vi "strip_path_multiple.vi"(8 "error in (no error)":errorcluster, 10 "number of strips":i32=1, 11 "path in":path) -> (0 "error out":errorcluster, 3 "path out":path)   [LabVIEW 2010]
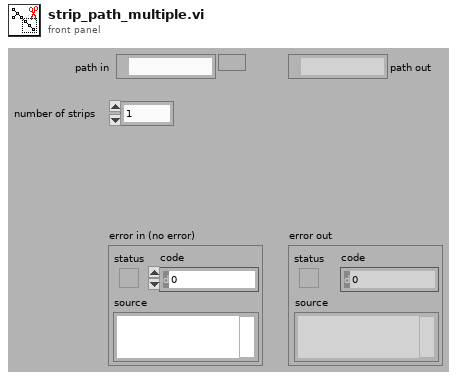
[diagram p1: front panel]
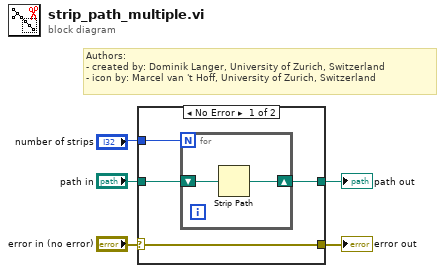
[diagram p0: block diagram]
diagram:
  # "Authors: \n- created by: Dominik Langer, University of Zurich, Switzerland\n- icon by: Marcel van 't Hoff, University of Zurich, Switzerland"
  n1 = case shown="No Error" "error in (no error)" {
    selector: "error in (no error)" -> [w7 w12]
    tunnel: "path in" -> [w9 w13]
    tunnel: [w8 w13] -> w3
    tunnel: [w7 w12] -> w2
    tunnel: "number of strips" -> [w6 _]
    frame No Error {
      n2 = for {
        N: w6 -> [_]
        shift-right: [w10] -> w8
        shift-left: w9 -> [w11]
        n3 = Strip Path(path=w11) -> (stripped path=w10:path)  [unwired: 1 out]
      }
    }
    frame Error {
    }
  }
  "error out" <- w2
  "path out" <- w3
